vi "Read and Modify HWS.vi"() -> ()   [LabVIEW 2013]
uses:
  <vilib>/Waveform/DWDTOps.llb/DWDT Digital to Boolean Array.vi
  <vilib>/Waveform/DWDTOps.llb/DWDT Boolean Array to Digital.vi
panel:
  out "USID and Command Read":bool[](array[boolean])
  out "Reg Address":bool[](array[boolean])
  out "Command Frame parity read":bool
  out "Data Frame Parity Read":bool
  out "Data Read":bool[](array[boolean])
  out "Data Frame Parity Read":bool[](array[boolean])
  out "Command Frame parity read":bool[](array[boolean])
  out "Register Readback":bool[](array[boolean])
  out "New Command Frame Parity to Write":bool
  out "New Data Frame Parity to Write":bool
  out "Match?":bool
  in  "Filename":string
  in  "Save file?":bool
  in  "New Address to Write":u8=21 format="%.0x"
  out "Data Read":u8=4 format="%.0b"
  out "Reg Address Read":u8=4 format="%.0x"
  in  "New Data to Write":u8=4 format="%.0b"
  in  "Starting HWS File":path=path "D:/San Jose/CK Lab/T Bench/CK-MC3-X1/Waveforms/RFFE7/LowPowerMode.hws"
  out "New  HWS File to Create":digitalwaveform(graph)
  out "HWS File Read":digitalwaveform(graph)
  # "FOR DEBUGGING:"
  # "i"
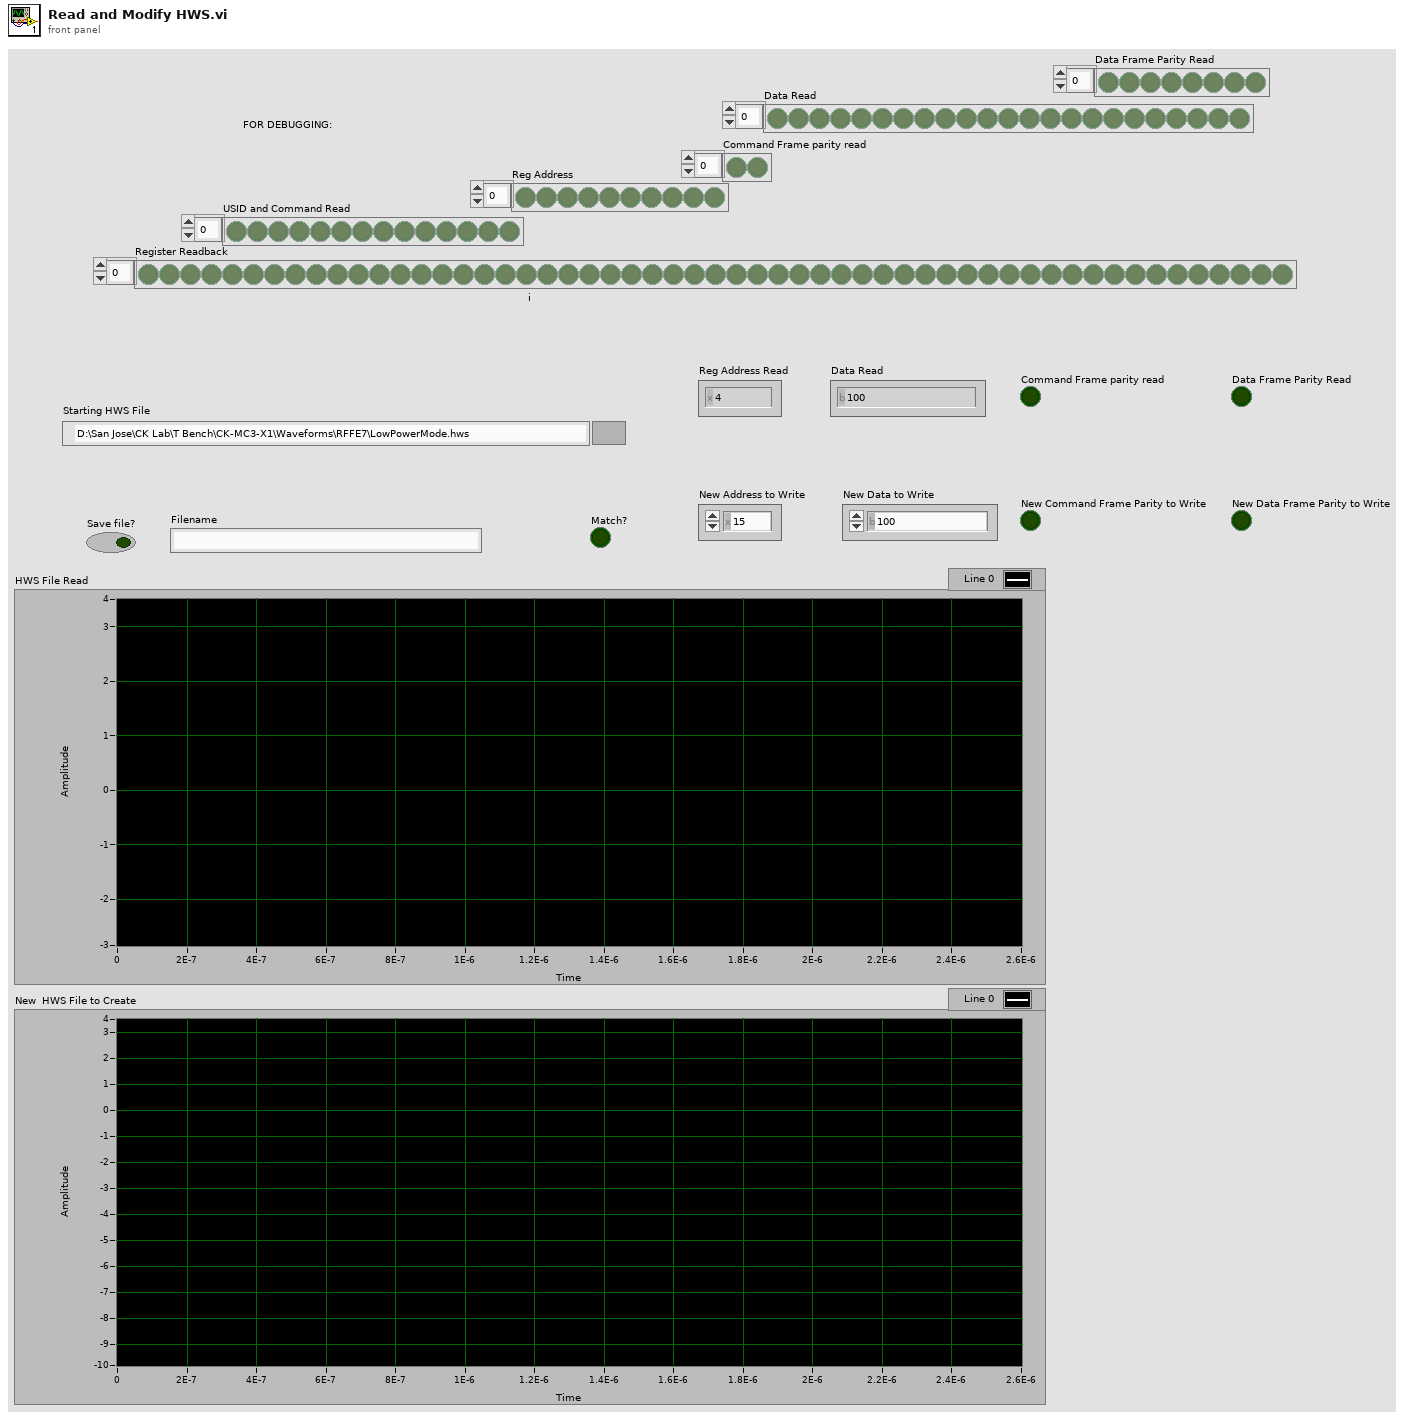
[diagram p1: front panel]
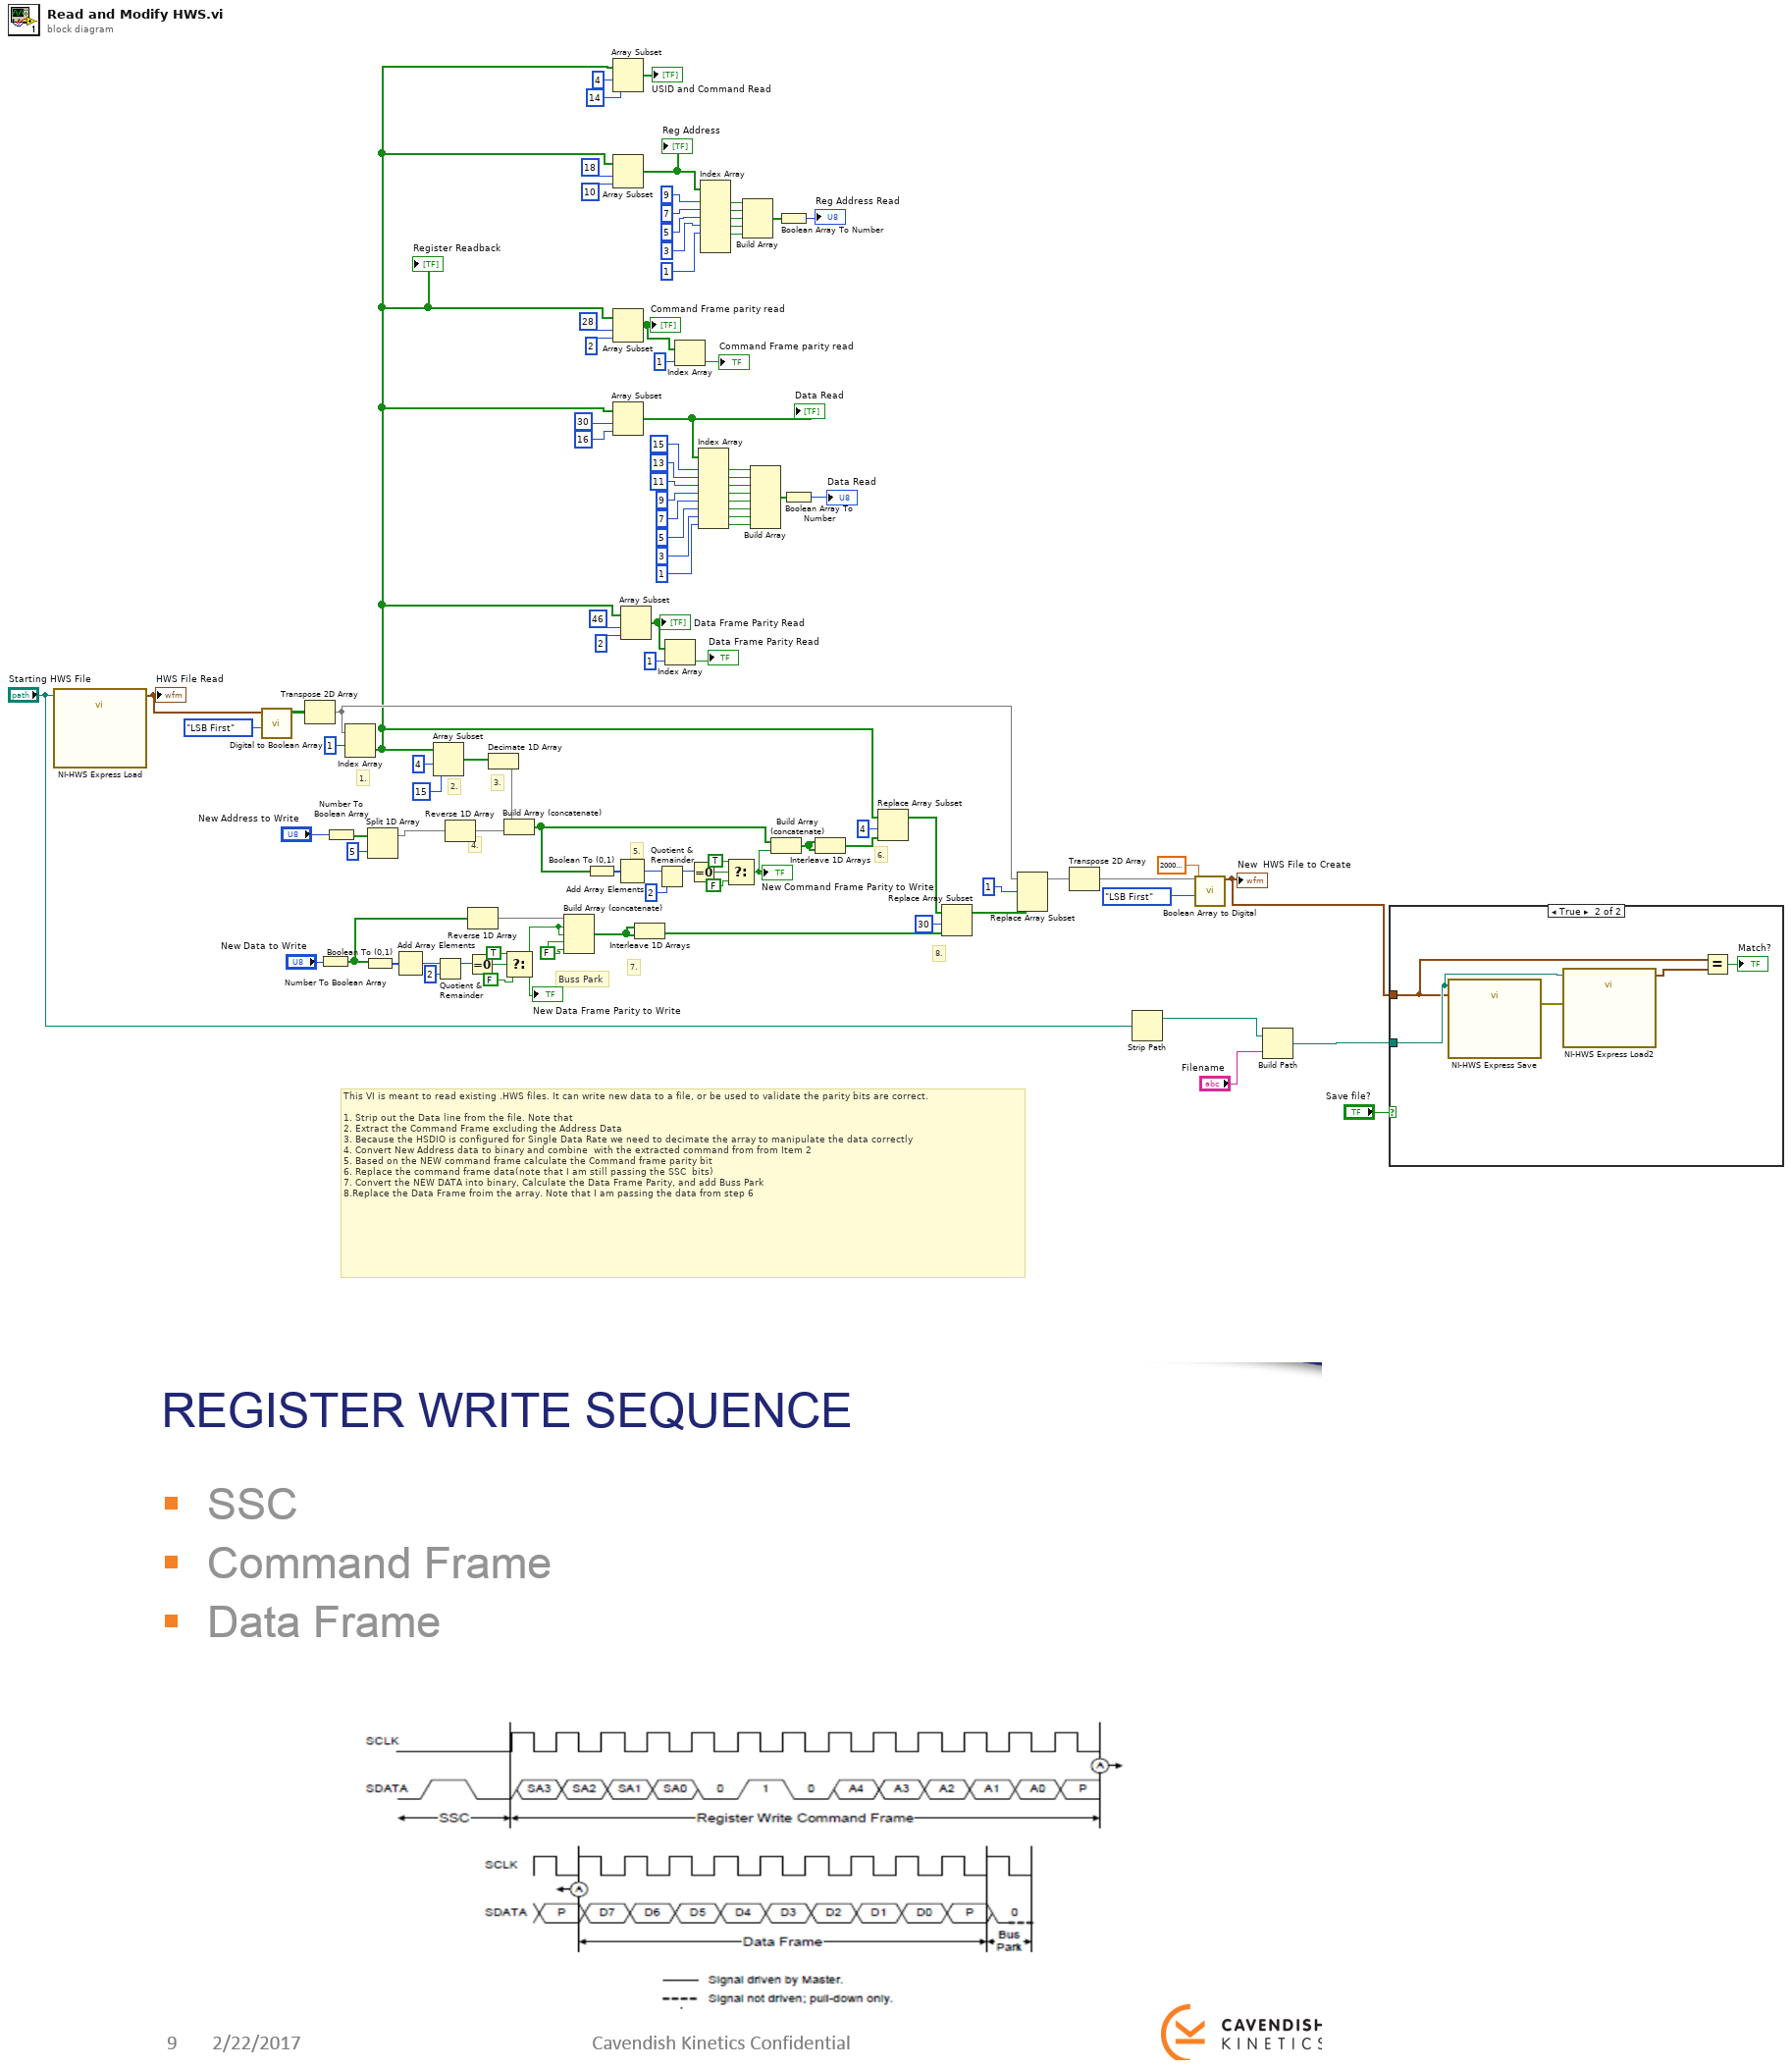
[diagram p0: block diagram]
diagram:
  w4 = FALSE ("element")
  # "6."
  # "This VI is meant to read existing .HWS files. It can write new data to a file, or be used to validate the parity bits are correct.\n\n1. Strip out the Data line from the file. Note that \n2. Extract the Command Frame excluding the Address Data\n3. Because the HSDIO is configured for Single Data Rate we need to decimate the array to manipulate the data correctly\n4. Convert New Address data to binary and combine  with the extracted command from from Item 2\n5. Based on the NEW command frame calculate the Command frame parity bit\n6. Replace the command frame data(note that I am still passing the SSC  bits)\n7. Convert the NEW DATA into binary, Calculate the Data Frame Parity, and add Buss Park\n8.Replace the Data Frame froim the array. Note that I am passing the data from step 6"
  # "8."
  # "7."
  # "5."
  # "4."
  # "3."
  # "2."
  # "1."
  # "Buss Park"
  n1 = call "NI-HWS Express Load"("file path"="Starting HWS File") -> ("LowPowerMode.hws"=w17:digitalwaveform)  [unwired: 9 in, 1 out]
  "HWS File Read" <- w17
  n2 = call-poly <vilib>:"Digital to Boolean Array.vi"("mode"=enum16{"LSB First", "MSB First"}."LSB First", "digital waveform"=w17) -> ("boolean array"=w103:bool[][])  [unwired: 8 in, 1 out]
  n3 = Transpose 2D Array(2D array=w103) -> (transposed array=w91:bool[][])
  n4 = Number To Boolean Array(number="New Data to Write") -> (Boolean array=w44:bool[])
  n5 = Number To Boolean Array(number="New Address to Write") -> (Boolean array=w41:bool[])
  n6 = Index Array(array=w91, index (row)=1) -> (element=w12:bool[])  [unwired: 1 in]
  "Register Readback" <- w12
  n7 = Boolean To (0,1)(Boolean=w44) -> (0, 1=w43:i16[])
  n8 = Split 1D Array(array=w41, index=5) -> (first subarray=w3:bool[])  [unwired: 1 out]
  n9 = Add Array Elements(numeric array=w43) -> (sum=w46:i16)
  n10 = Array Subset(array=w12, index=4, length=15) -> (w19:bool[])
  n11 = Quotient & Remainder(x=w46, y=i16 2) -> (x-y*floor(x/y)=w42:i16)  [unwired: 1 out]
  n12 = Reverse 1D Array(array=w3) -> (reversed array=w2:bool[])
  n13 = Equal To 0?(x=w42) -> (x = 0?=w96:bool)
  n14 = Reverse 1D Array(array=w44) -> (reversed array=w93:bool[])
  n15 = Decimate 1D Array(w19) -> (w16:bool[])  [unwired: 1 out]
  n16 = Build Array (concatenate)(w16, w2) -> (w1:bool[])
  n17 = Select(t=TRUE, s=w96, f=FALSE) -> (s? t:f=w5:bool)
  "New Data Frame Parity to Write" <- w5
  n18 = Build Array (concatenate)(w93, w5, w5, w4, w4) -> (w92:bool[])
  n19 = Boolean To (0,1)(Boolean=w1) -> (0, 1=w15:i16[])
  n20 = Array Subset(array=w12, index=4, length=14) -> (→"USID and Command Read":bool[])
  n21 = Array Subset(array=w12, index=18, length=10) -> (w86:bool[])
  "Reg Address" <- w86
  n22 = Array Subset(array=w12, index=28, length=2) -> (w30:bool[])
  "Command Frame parity read" <- w30
  n23 = Array Subset(array=w12, index=30, length=16) -> (w72:bool[])
  "Data Read" <- w72
  n24 = Add Array Elements(numeric array=w15) -> (sum=w22:i16)
  n25 = Array Subset(array=w12, index=46, length=2) -> (w34:bool[])
  "Data Frame Parity Read" <- w34
  n26 = Interleave 1D Arrays(w92, w92) -> (w7:bool[])
  n27 = Quotient & Remainder(x=w22, y=i16 2) -> (x-y*floor(x/y)=w20:i16)  [unwired: 1 out]
  n28 = Index Array(array=w34, index=1) -> (element=→"Data Frame Parity Read":bool)
  n29 = Index Array(array=w30, index=1) -> (element=→"Command Frame parity read":bool)
  n30 = Equal To 0?(x=w20) -> (x = 0?=w25:bool)
  n31 = Index Array(array=w72, index #1=15 ("index"), index #2=13 ("index"), index #3=11 ("index"), index #4=9 ("index"), index #5=7 ("index"), index #6=5 ("index"), index #7=3 ("index"), index #8=1 ("index")) -> (element #1=w62:bool, element #2=w61:bool, element #3=w60:bool, element #4=w59:bool, element #5=w58:bool, element #6=w57:bool, element #7=w56:bool, element #8=w52:bool)
  n32 = Index Array(array=w86, index #1=9 ("index"), index #2=7 ("index"), index #3=5 ("index"), index #4=3 ("index"), index #5=1 ("index")) -> (element #1=w80:bool, element #2=w79:bool, element #3=w78:bool, element #4=w77:bool, element #5=w76:bool)  [unwired: 2 in, 2 out]
  n33 = Select(t=TRUE, s=w25, f=FALSE) -> (s? t:f=w14:bool)
  "New Command Frame Parity to Write" <- w14
  n34 = Build Array(w80, w79, w78, w77, w76) -> (w75:bool[])
  n35 = Build Array(w62, w61, w60, w59, w58, w57, w56, w52) -> (w64:bool[])
  n36 = Build Array (concatenate)(w1, w14) -> (w13:bool[])
  n37 = Boolean Array To Number(Boolean array=w75) -> (number=→"Reg Address Read":u8)
  n38 = Boolean Array To Number(Boolean array=w64) -> (number=→"Data Read":u8)
  n39 = Interleave 1D Arrays(w13, w13) -> (w10:bool[])
  n40 = Replace Array Subset(array=w12, new element=w10, index=4) -> (w8:bool[])
  n41 = Replace Array Subset(array=w8, new element=w7, index=30) -> (w6:bool[])
  n42 = Replace Array Subset(array=w91, new element=w6, index (row)=1) -> (w89:bool[][])  [unwired: 1 in]
  n43 = Transpose 2D Array(2D array=w89) -> (transposed array=w102:bool[][])
  n44 = Strip Path(path="Starting HWS File") -> (stripped path=w54:path)  [unwired: 1 out]
  n45 = call-poly <vilib>:"Boolean Array to Digital.vi"("mode"=enum16{"LSB First", "MSB First"}."LSB First", "sample rate"=20000000.0, "boolean array"=w102) -> ("digital waveform"=w18:digitalwaveform)  [unwired: 7 in, 1 out]
  "New  HWS File to Create" <- w18
  n46 = Build Path(base path=w54, name or relative path="Filename") -> (appended path=w49:path)
  n47 = case shown="True" "Save file?" {
    tunnel: w18 -> [_ w106]
    tunnel: w49 -> [_ w108]
    frame False {
    }
    frame True {
      n48 = call "NI-HWS Express Save"("digital waveform"=w106, "file path"=w108) -> ("error out"=w109:errorcluster)  [unwired: 9 in]
      n49 = call "NI-HWS Express Load2"("error in"=w109, "file path"=w108) -> ("LowPowerMode.hws"=w107:digitalwaveform)  [unwired: 8 in, 1 out]
      n50 = Equal?(x=w106, y=w107) -> (x = y?=→"Match?":bool)
    }
  }
